vi "Load Motion Profile.vi"(3 "AUTO START POSITION":string) -> ()   [LabVIEW 2019]
uses:
  <vilib>/Rock Robotics/WPI/ThirdParty/Phoenix-LabVIEW/Motor Controller/Controls/CTRE_Phoenix_MotorControl_MotionProfileTrajectoryPoint.ctl
  RoboRIO/Global Data.vi
  <vilib>/Utility/file.llb/Read Delimited Spreadsheet (DBL).vi
  <vilib>/Rock Robotics/WPI/ThirdParty/Phoenix-LabVIEW/Motor Controller/Closed Loop/Motion Profile/CTRE_Phoenix_MotorControl_BufferedTrajectoryPointStream_WriteAll.vi
  RoboRIO/Refnums.vi
panel:
  in  "File Path":path=path "/home/lvuser/paths"
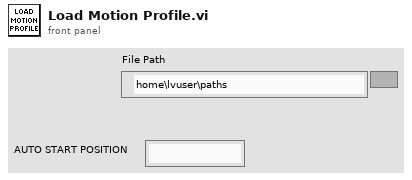
[diagram p1: front panel]
types:
  T1 = typedef "CTRE_Phoenix_MotorControl_MotionProfileTrajectoryPoint.ctl" = cluster{"Position":dbl, "Velocity":dbl, "Arbitrary Feed Forward":dbl, "Auxiliary Position":dbl, "Auxiliary Velocity":dbl, "Auxiliary Arbitrary Feed Forward":dbl, "Profile Slot Select":i32, "Auxiliary Profile Slot Select":i32, "isLastPoint?":bool, "Zero Position?":bool, "durationMs":u32, "Use Aux PID?":bool}
  T2 = typedef "CTRE_Phoenix_MotorControl_BufferedTrajectoryPointStream_DeviceRef.ctl" = cluster{"Handle":u64, "Library Path":path}
  T3 = cluster{"[0]":T2, "[1]":T2, "[2]":T2, "[3]":T2, "[4]":T2, "[5]":T2, "[6]":T2, "[7]":T2, "[8]":T2}
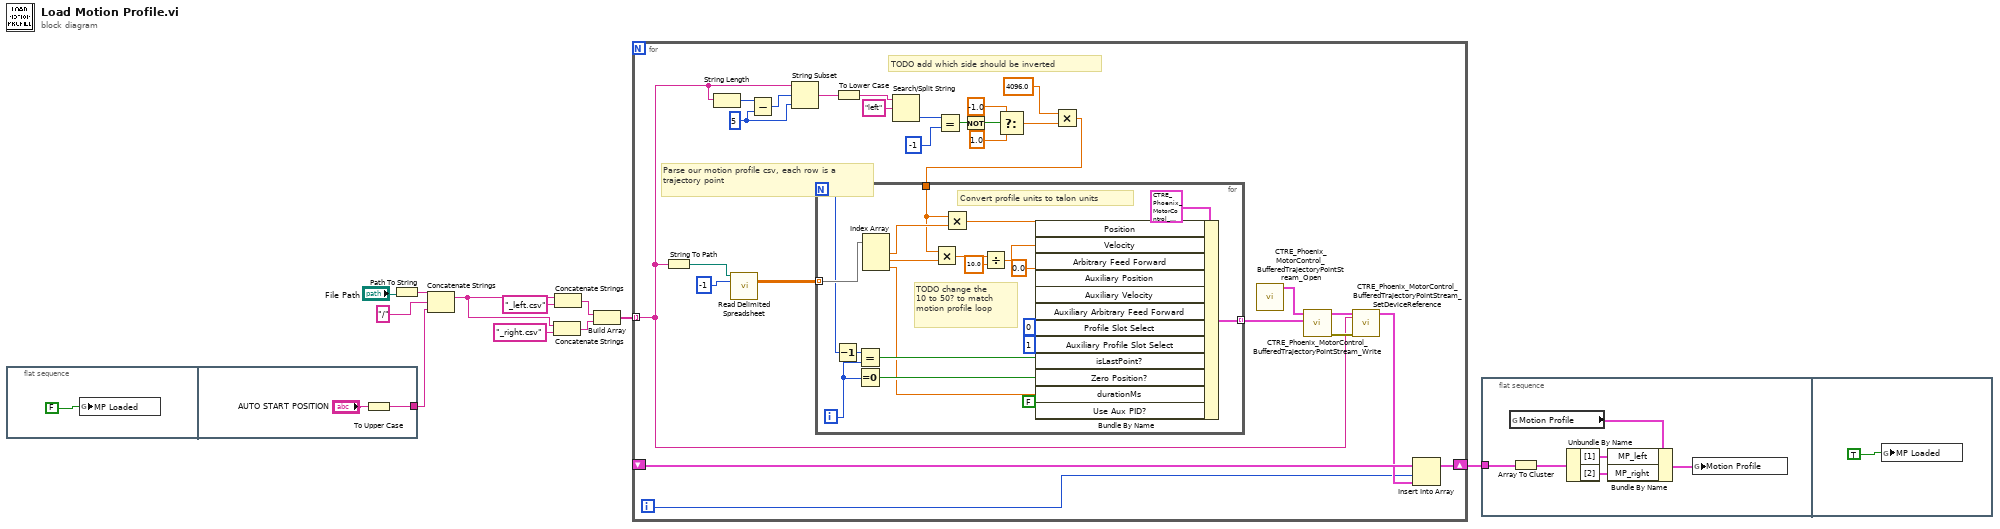
[diagram p0: block diagram]
diagram:
  n1 = flat-sequence {
    tunnel: [w13] -> w1
    frame #0 {
      n2 = global write "Global Data.vi" "MP Loaded"(FALSE) -> ()
    }
    frame #1 {
      n3 = To Upper Case(1:"AUTO START POSITION") -> (0:w13:string)
    }
  }
  n4 = Path To String(path="File Path") -> (string=w10:string)
  n5 = Concatenate Strings(w10, "/" ("string"), w1) -> (w4:string)
  n6 = Concatenate Strings(w4, "_right.csv" ("string")) -> (w5:string)
  n7 = Concatenate Strings(w4, "_left.csv" ("string")) -> (w8:string)
  n8 = Build Array(w8, w5) -> (w3:string[])
  n9 = for {
    tunnel: w3 -> [w21] mode=indexing
    shift-right: [w17] -> w2
    shift-left: _ -> [w20]
    i -> [w18]
    w32 = 5 ("y")
    # "TODO add which side should be inverted"
    # "Parse our motion profile csv, each row is a trajectory point"
    n10 = String To Path(string=w21) -> (path=w23:path)
    n11 = String Length(string=w21) -> (length=w34:i32)
    n12 = call-poly <vilib>:"Read Delimited Spreadsheet.vi"("file path (dialog if empty)"=w23, "number of rows (all:-1)"=-1) -> ("all rows"=w40:dbl[][])  [unwired: 8 in, 5 out]
    n13 = Subtract(x=w34, y=w32) -> (x-y=w33:i32)
    n14 = String Subset(string=w21, offset (0)=w33, length (rest)=w32) -> (substring=w31:string)
    n15 = To Lower Case(string=w31) -> (all lower case string=w30:string)
    n16 = Search/Split String(string=w30, search string/char (-)="left") -> (offset of match=w28:i32)  [unwired: 1 in, 2 out]
    n17 = Equal?(x=w28, y=-1) -> (x = y?=w26:bool)
    n18 = Not(x=w26) -> (.not. x?=w25:bool)
    n19 = Select(t=-1.0, s=w25, f=1.0) -> (s? t:f=w24:dbl)
    n20 = Multiply(x=4096.0, y=w24) -> (x*y=w22:dbl)
    n21 = for {
      N -> [w54]
      tunnel: w40 -> [w60] mode=indexing
      tunnel: [w50] -> w39 mode=indexing
      tunnel: w22 -> [w42]
      i -> [w53]
      w59 = 0.0 ("Arbitrary Feed Forward")
      # "TODO change the \n10 to 50? to match \nmotion profile loop"
      # "Convert profile units to talon units"
      n22 = Decrement(x=w54) -> (x-1=w55:i32)
      n23 = Equal?(x=w55, y=w53) -> (x = y?=w56:bool)
      n24 = Equal To 0?(x=w53) -> (x = 0?=w52:bool)
      n25 = Index Array(array=w60) -> (element #1=w48:dbl, element #2=w44:dbl, element #3=w49:dbl)  [unwired: 3 in]
      n26 = Multiply(x=w42, y=w44) -> (x*y=w46:dbl)
      n27 = Multiply(x=w42, y=w48) -> (x*y=w47:dbl)
      n28 = Divide(x=w46, y=10.0) -> (x/y=w43:dbl)
      n29 = Bundle By Name(cluster=T1 {"Position"=0.0, "Velocity"=0.0, "Arbitrary Feed Forward"=0.0, "Auxiliary Position"=0.0, "Auxiliary Velocity"=0.0, "Auxiliary Arbitrary Feed Forward"=0.0, "Profile Slot Select"=0, "Auxiliary Profile Slot Select"=0, "isLastPoint?"=FALSE, "Zero Position?"=FALSE, "durationMs"=0, "Use Aux PID?"=FALSE} ("Trajectory Point"), "Position"=w47, "Velocity"=w43, "Arbitrary Feed Forward"=w59, "Auxiliary Position"=w59, "Auxiliary Velocity"=w59, "Auxiliary Arbitrary Feed Forward"=w59, "Profile Slot Select"=0, "Auxiliary Profile Slot Select"=1, "isLastPoint?"=w56, "Zero Position?"=w52, "durationMs"=w49, "Use Aux PID?"=FALSE) -> (w50:T1)
    }
    n30 = call <vilib>:"CTRE_Phoenix_MotorControl_BufferedTrajectoryPointStream_Open.vi"() -> ("BufferedTrajectoryPointStream_DevRef"=w38:T2)  [unwired: 10 in, 1 out]
    n31 = call-poly <vilib>:"CTRE_Phoenix_MotorControl_BufferedTrajectoryPointStream_Write.vi"("Motion Profile Trajectory Point Array"=w39, "BufferedTrajectoryPointStream_DevRef"=w38) -> ("error out"=w36:errorcluster, "BufferedTrajectoryPointStream_DevRef"=w37:T2)  [unwired: 8 in]
    n32 = call <vilib>:"CTRE_Phoenix_MotorControl_BufferedTrajectoryPointStream_SetDeviceReference.vi"("error in (no error)"=w36, "refnum name"=w21, "BufferedTrajectoryPointStream_DevRef"=w37) -> ("BufferedTrajectoryPointStream_DevRef"=w19:T2)  [unwired: 7 in, 1 out]
    n33 = Insert Into Array(array=w20, index=w18, new element=w19) -> (w17:T2[])
  }
  n34 = flat-sequence {
    tunnel: w2 -> [w67]
    frame #0 {
      n35 = global read "Refnums.vi" "Motion Profile"() -> (w65:cluster{"MP_left":T2, "MP_right":T2})
      n36 = Array To Cluster(array=w67) -> (cluster=w66:T3)
      n37 = Unbundle By Name(w66) -> ("[1]"=w64:T2, "[2]"=w63:T2)
      n38 = Bundle By Name(cluster=w65, "MP_left"=w64, "MP_right"=w63) -> (w62:cluster{"MP_left":T2, "MP_right":T2})
      n39 = global write "Refnums.vi" "Motion Profile"(w62) -> ()
    }
    frame #1 {
      n40 = global write "Global Data.vi" "MP Loaded"(TRUE) -> ()
    }
  }
